vi "serial key 생성기.vi"() -> ()   [LabVIEW 2014]
panel:
  in  "?":bool
  out "serial number":string
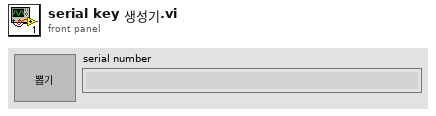
[diagram p1: front panel]
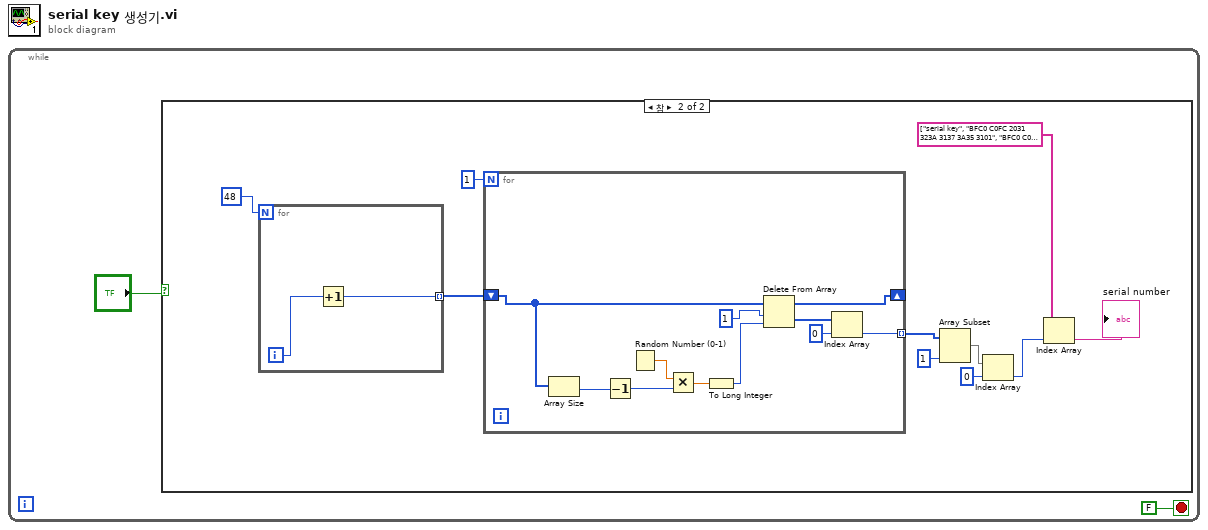
[diagram p0: block diagram]
diagram:
  n1 = while {
    stop <- FALSE stop-if-true
    n2 = case shown="참" "?" {
      frame False {
      }
      frame True {
        n3 = for {
          N: 48 -> [_]
          tunnel: [w24] -> w11 mode=indexing
          i -> [w25]
          n4 = Increment(x=w25) -> (x+1=w24:i32)
        }
        n5 = for {
          N: 1 -> [_]
          shift-right: [w23] -> _
          shift-left: w11 -> [w18]
          tunnel: [w13] -> w10 mode=indexing
          n6 = Array Size(array=w18) -> (size(s)=w19:i32)
          n7 = Decrement(x=w19) -> (x-1=w17:i32)
          n8 = Random Number (0-1)() -> (number: 0 to 1=w20:dbl)
          n9 = Multiply(x=w20, y=w17) -> (x*y=w16:dbl)
          n10 = To Long Integer(number=w16) -> (32bit integer=w15:i32)
          n11 = Delete From Array(array=w18, length=1, index=w15) -> (deleted portion=w14:i32[], array with subset deleted=w23:i32[])
          n12 = Index Array(array=w14, index=0 ("인덱스")) -> (element=w13:i32)
        }
        n13 = Array Subset(array=w10, length=1 ("길이")) -> (w7:i32[])  [unwired: 1 in]
        n14 = Index Array(array=w7, index=0 ("인덱스")) -> (element=w5:i32)
        n15 = Index Array(array=string[] ["serial key", "BFC0 C0FC 2031 323A 3137 3A35 3101", "BFC0 C0FC 2031 323A 3138 3A30 3902", "BFC0 C0FC 2031 323A 3139 3A30 3903", "BFC0 C0FC 2031 323A 3230 3A30 3904", "BFC0 C0FC 2031 323A 3231 3A30 3905", "BFC0 C0FC 2031 323A 3232 3A30 3906", "BFC0 C0FC 2031 323A 3233 3A30 3907", "BFC0 C0FC 2031 323A 3234 3A30 3908", "BFC0 C0FC 2031 323A 3235 3A30 3909", "BFC0 C0FC 2031 323A 3236 3A30 3910", "BFC0 C0FC 2031 323A 3237 3A30 3911", "BFC0 C0FC 2031 323A 3238 3A30 3912", "BFC0 C0FC 2031 323A 3239 3A30 3913", "BFC0 C0FC 2031 323A 3036 3A33 3214", "BFC0 C0FC 2031 323A 3037 3A33 3215", "BFC0 C0FC 2031 323A 3038 3A33 3216", "BFC0 C0FC 2031 323A 3038 3A33 3217", "BFC0 C0FC 2031 323A 3039 3A33 3218", "BFC0 C0FC 2031 323A 3039 3A35 3019", "BFC0 C0FC 2031 323A 3130 3A35 3020", "BFC0 C0FC 2031 323A 3131 3A35 3121", "BFC0 C8C4 2031 313A 3536 3A33 3222", "BFC0 C8C4 2031 313A 3537 3A33 3223", "BFC0 C8C4 2031 313A 3538 3A33 3224", "BFC0 C8C4 2031 313A 3539 3A33 3225", "BFC0 C0FC 2031 323A 3030 3A33 3226", "BFC0 C0FC 2031 323A 3031 3A33 3227", "BFC0 C0FC 2031 323A 3032 3A33 3228", "BFC0 C0FC 2031 323A 3033 3A33 3229", "BFC0 C0FC 2031 323A 3034 3A33 3230", "BFC0 C0FC 2031 323A 3035 3A33 3231", "BFC0 C0FC 2031 323A 3036 3A33 3232", "BFC0 C0FC 2031 323A 3037 3A33 3233", "BFC0 C0FC 2031 323A 3038 3A33 3234", "BFC0 C0FC 2033 3A34 373A 3031 0035 ", "BFC0 C0FC 2033 3A34 383A 3234 0036", "BFC0 C0FC 2033 3A34 393A 3132 0037", "BFC0 C0FC 2033 3A35 303A 3534 0038", "BFC0 C0FC 2033 3A35 313A 3231 0039 ", "BFC0 C0FC 2033 3A35 323A 3333 0040 ", "BFC0 C0FC 2033 3A35 333A 3030 0041", "BFC0 C0FC 2033 3A35 343A 3432 0042", "BFC0 C0FC 2033 3A35 353A 3431 0043", "BFC0 C0FC 2033 3A35 363A 3131 0044", "BFC0 C0FC 2033 3A35 373A 3239 0045", "BFC0 C0FC 2033 3A35 383A 3539 0046", "BFC0 C0FC 2033 3A35 393A 3533 0047", "BFC0 C0FC 2034 3A30 303A 3430 0048 "] ("출력 배열"), index=w5) -> (element=→"serial number":string)
      }
    }
  }
